vi "Cut.vi"(2 "Image":i32[][](array[numeric]), 4 "Width":i32) -> (5 "Maximum":i32, 6 "Y Cut":i32[](array[numeric]), 7 "X Cut":i32[](array[numeric]))   [LabVIEW 2009]
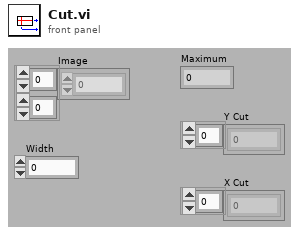
[diagram p1: front panel]
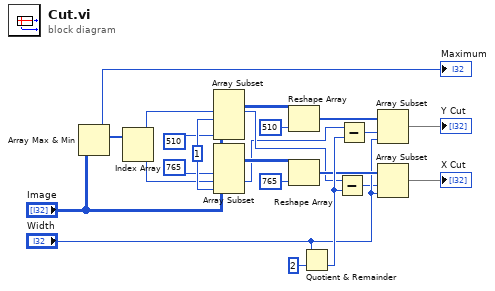
[diagram p0: block diagram]
diagram:
  w14 = 1
  n1 = Array Max & Min(array="Image") -> (max value=→"Maximum":i32, max index (indices)=w1:i32[])  [unwired: 2 out]
  n2 = Index Array(array=w1) -> (element #1=w3:i32, element #2=w2:i32)  [unwired: 2 in]
  n3 = Array Subset(array="Image", index (row)=w3, length (row)=w14, length (col)=510) -> (w5:i32[][])  [unwired: 1 in]
  n4 = Array Subset(array="Image", length (row)=765, index (col)=w2, length (col)=w14) -> (w4:i32[][])  [unwired: 1 in]
  n5 = Reshape Array(w5, 510) -> (w16:i32[])
  n6 = Reshape Array(w4, 765) -> (w15:i32[])
  n7 = Quotient & Remainder(x="Width", y=2) -> (floor(x/y)=w21:i32)  [unwired: 1 out]
  n8 = Subtract(x=w3, y=w21) -> (x-y=w12:i32)
  n9 = Subtract(x=w2, y=w21) -> (x-y=w11:i32)
  n10 = Array Subset(array=w16, index=w11, length="Width") -> (→"Y Cut":i32[])
  n11 = Array Subset(array=w15, index=w12, length="Width") -> (→"X Cut":i32[])
